vi "NiFPGA Get P2P FIFO Endpoint.vi"(8 "error in (no error)":errorcluster, 10 "FIFO":u32, 11 "Session":u32) -> (0 "error out":errorcluster, 1 "Endpoint":u32, 3 "Session Out":u32)   [LabVIEW 2010, in "FPGA Interface Wrapper.lvlib"]
doc: "Gets an endpoint reference to a peer-to-peer FIFO."
uses:
  <userlib>/_FPGA Interface Advanced Tools/FPGA Interface Wrapper/FPGA Interface Wrapper.lvlib
  NiFpga.dll
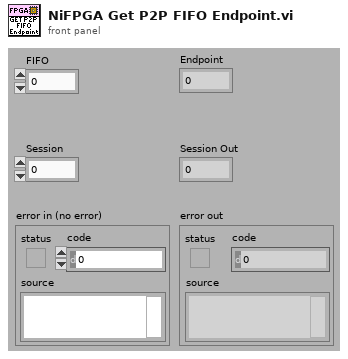
[diagram p1: front panel]
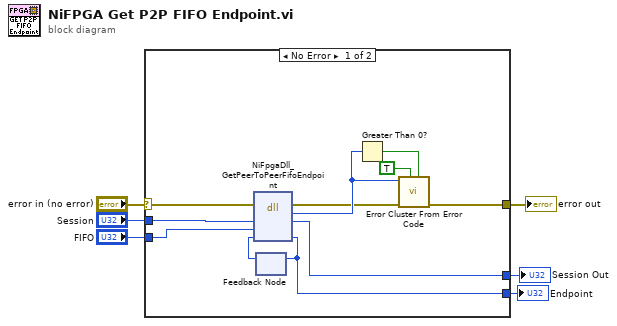
[diagram p0: block diagram]
diagram:
  n1 = case shown="No Error" "error in (no error)" {
    selector: "error in (no error)" -> [w17 w18]
    tunnel: [w7 w18] -> w5
    tunnel: "Session" -> [w16 w19]
    tunnel: [w15 w19] -> w3
    tunnel: "FIFO" -> [w14 _]
    tunnel: [w12 _] -> w1
    frame No Error {
      n2 = feedback #1() -> (w13:u32)  [unwired: 1 in]
      n3 = dll-call lib="NiFpga.dll" fn="NiFpgaDll_GetPeerToPeerFifoEndpoint"(error in=w17, "Session"=w16, "FIFO"=w14, "Endpoint"=w13) -> (error out=w8:errorcluster, "Status"=w9:i32, "Session"=w15:u32, "Endpoint"=w12:u32)  [unwired: 3 in, 1 out]
      n4 = feedback-in #1(w12) -> ()
      n5 = Greater Than 0?(x=w9) -> (x > 0?=w10:bool)
      n6 = call <vilib>:"Error Cluster From Error Code.vi"("is warning? (False)"=w10, "show call chain? (False)"=TRUE, "error in (no error)"=w8, "error code (0)"=w9) -> ("error out"=w7:errorcluster)  [unwired: 5 in]
    }
    frame Error {
    }
  }
  "error out" <- w5
  "Session Out" <- w3
  "Endpoint" <- w1
